vi "Remove System.vi"(8 "error in (no error)":errorcluster, 11 "Manager in":refnum<class "Manager.lvclass">) -> (0 "error out":errorcluster, 3 "Manager out":refnum<class "Manager.lvclass">)   [LabVIEW 2012, in "Manager.lvlib" / "Manager.lvclass"]
uses:
  Manager.lvclass
  Manager.lvclass/Manager.ctl
  <vilib>/ActorFramework/Actor/Actor.lvclass/Actor.ctl
  <vilib>/ActorFramework/Message Enqueuer/Message Enqueuer.lvclass/Message Enqueuer.ctl
  Write Control Systems.vi
  Read System Ring Refnum.vi
  Read Control Systems.vi
  Read Remove Button Refnum.vi
  <vilib>/ActorFramework/Message Enqueuer/Init from Existing Queue.vi
  <vilib>/ActorFramework/Message Enqueuer/Enqueue.vi
  <vilib>/ActorFramework/Stop Msg/Send Emergency Stop.vi
  <vilib>/ActorFramework/Message Enqueuer/Enqueue Critical.vi
  <vilib>/ActorFramework/Message Priority Queue/Priority Enqueue.vi
  <vilib>/ActorFramework/Message Enqueuer/Message Enqueuer.lvclass
  Manager Messages/Update SubPanel Msg/Update SubPanel Msg.lvclass
  <vilib>/ActorFramework/Stop Msg/Stop Msg.lvclass
  <vilib>/ActorFramework/Actor/Actor.lvclass
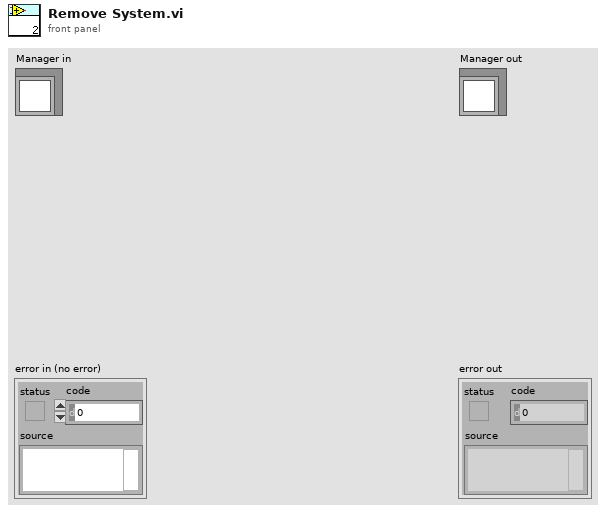
[diagram p1: front panel]
types:
  T1 = cluster{"Bioreactor Queue":refnum<class "Message Enqueuer.lvclass">, "Time Protocol Queue":refnum<class "Message Enqueuer.lvclass">, "Python Protocol Queue":refnum<class "Message Enqueuer.lvclass">, "Name":string}[]
  T2 = cluster{"Bioreactor Queue":refnum<class "Message Enqueuer.lvclass">, "Time Protocol Queue":refnum<class "Message Enqueuer.lvclass">, "Python Protocol Queue":refnum<class "Message Enqueuer.lvclass">, "Name":string}
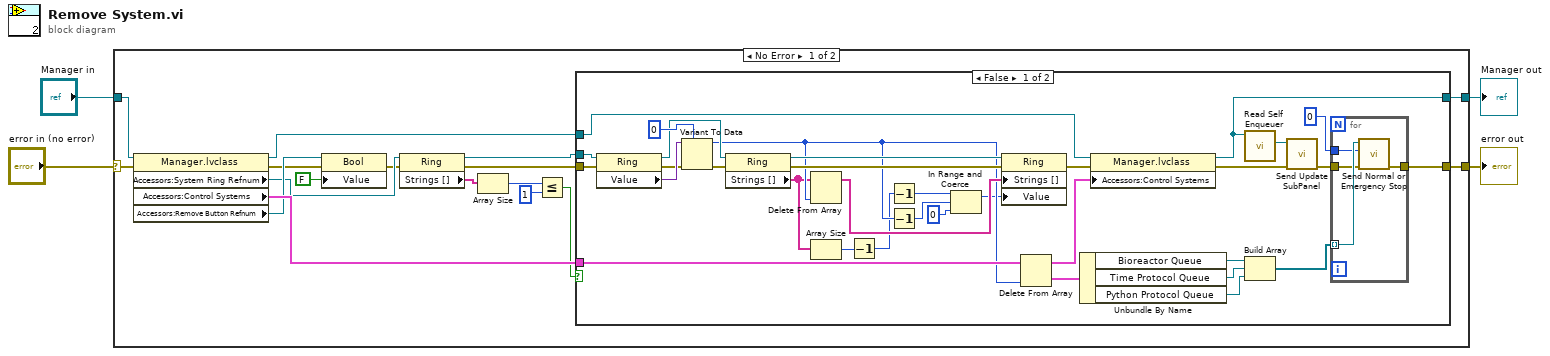
[diagram p0: block diagram]
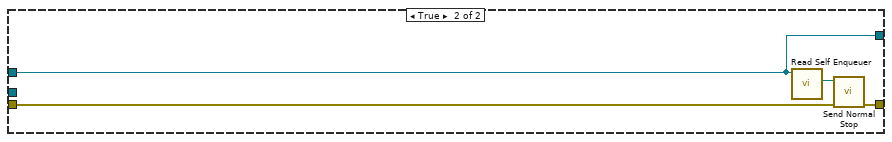
[diagram p2: hidden frame]
diagram:
  n1 = case shown="No Error" "error in (no error)" {
    selector: "error in (no error)" -> [w21 w64]
    tunnel: [w19 w64] -> w3
    tunnel: [w16 w63] -> w1
    tunnel: "Manager in" -> [w20 w63]
    frame No Error {
      n2 = property class="Manager.lvclass"(reference=w20, error in=w21) -> (reference out=w17:refnum<class "Manager.lvclass">, error out=w13:errorcluster, "Accessors:System Ring Refnum"=w12:refnum<vi>, "Accessors:Control Systems"=w18:T1, "Accessors:Remove Button Refnum"=w15:refnum<vi>)
      n3 = property class="Bool"(reference=w15, error in=w13, "Value"=FALSE) -> (error out=w10:errorcluster)  [unwired: 1 out]
      n4 = property class="Ring"(reference=w12, error in=w10) -> (reference out=w11:refnum<vi>, error out=w9:errorcluster, "Strings []"=w8:string[])
      n5 = Array Size(array=w8) -> (size(s)=w5:i32)
      n6 = Less Or Equal?(x=w5, y=1) -> (x <= y?=w6:bool)
      n7 = case shown="False" w6 {
        tunnel: [w39 w60] -> w19
        tunnel: w18 -> [w38 _]
        tunnel: w17 -> [w36 w59]
        tunnel: [w35 w59] -> w16
        tunnel: w11 -> [w31 _]
        tunnel: w9 -> [w30 w61]
        frame False {
          n8 = property class="Ring"(reference=w31, error in=w30) -> (reference out=w50:refnum<vi>, error out=w52:errorcluster, "Value"=w54:variant)
          n9 = Variant To Data(error in=w52, type=0, Variant=w54) -> (data=w29:i32, error out=w51:errorcluster)
          n10 = property class="Ring"(reference=w50, error in=w51) -> (reference out=w48:refnum<vi>, error out=w47:errorcluster, "Strings []"=w24:string[])
          n11 = Delete From Array(array=w24, index=w29) -> (array with subset deleted=w49:string[])  [unwired: 1 in, 1 out]
          n12 = Array Size(array=w24) -> (size(s)=w23:i32)
          n13 = Decrement(x=w23) -> (x-1=w28:i32)
          n14 = Decrement(x=w28) -> (x-1=w22:i32)
          n15 = Decrement(x=w29) -> (x-1=w26:i32)
          n16 = In Range and Coerce(upper limit=w22, x=w26, lower limit=0) -> (coerced(x)=w25:i32)  [unwired: 1 out]
          n17 = property class="Ring"(reference=w48, error in=w47, "Strings []"=w49, "Value"=w25) -> (error out=w34:errorcluster)  [unwired: 1 out]
          n18 = Delete From Array(array=w38, index=w29) -> (deleted portion=w37:T2, array with subset deleted=w32:T1)  [unwired: 1 in]
          n19 = Unbundle By Name(w37) -> ("Bioreactor Queue"=w46:refnum<class "Message Enqueuer.lvclass">, "Time Protocol Queue"=w45:refnum<class "Message Enqueuer.lvclass">, "Python Protocol Queue"=w44:refnum<class "Message Enqueuer.lvclass">)
          n20 = property class="Manager.lvclass"(reference=w36, error in=w34, "Accessors:Control Systems"=w32) -> (reference out=w35:refnum<class "Manager.lvclass">, error out=w33:errorcluster)
          n21 = call <vilib>:"Read Self Enqueuer.vi"("Actor"=w35) -> ("Self Enqueuer"=w41:refnum<class "Message Enqueuer.lvclass">)  [unwired: 10 in]
          n22 = Build Array(w46, w45, w44) -> (w43:refnum<class "Message Enqueuer.lvclass">[])
          n23 = call "Send Update SubPanel.vi"("error in (no error)"=w33, "Message Enqueuer"=w41) -> ("error out"=w40:errorcluster)  [unwired: 8 in, 1 out]
          n24 = for {
            tunnel: w43 -> [w58] mode=indexing
            tunnel: 0 ("final error code") -> [w57]
            tunnel: [w56] -> w39
            tunnel: w40 -> [w55]
            n25 = call <vilib>:"Send Normal or Emergency Stop.vi"("error in (no error)"=w55, "final error code"=w57, "Message Enqueuer"=w58) -> ("error out"=w56:errorcluster)  [unwired: 8 in]
          }
        }
        frame True {
          n26 = call <vilib>:"Read Self Enqueuer.vi"("Actor"=w59) -> ("Self Enqueuer"=w62:refnum<class "Message Enqueuer.lvclass">)  [unwired: 10 in]
          n27 = call <vilib>:"Send Normal Stop.vi"("error in (no error)"=w61, "Message Enqueuer"=w62) -> ("error out"=w60:errorcluster)  [unwired: 9 in]
        }
      }
    }
    frame Error {
    }
  }
  "error out" <- w3
  "Manager out" <- w1
